vi "Module Template Configuraton Extractor API.vi"(8 "error constant":errorcluster, 11 "data value reference":refnum<data-value>) -> (0 "error out":errorcluster, 3 "Application Config":T1)   [LabVIEW 2021, in "Configuration.lvlib"]
doc: "This method extracts is a Poliphormic method used to read each module configuration."
uses:
  Imposible_Snake_v2/LVApp/Architecture/Modules/Configuration/Configuration.lvlib
  Application/App Configuration.ctl
  Imposible_Snake_v2/LVApp/Modules/Sound Manager/Typedefs/Config.ctl
  Imposible_Snake_v2/LVApp/Modules/Sound Manager/Sound Manager.lvlib
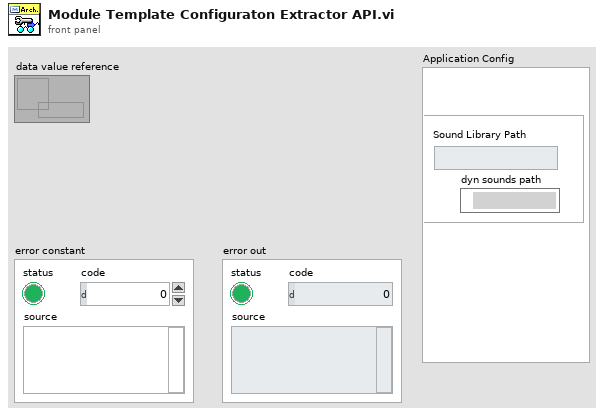
[diagram p1: front panel]
types:
  T1 = typedef "Application.lvclass/App Configuration.ctl" = cluster{"Sound Manager Config":T2}
  T2 = typedef "Sound Manager.lvlib/Config.ctl" = cluster{"Sound Library Path":path, "dyn sounds path":path}
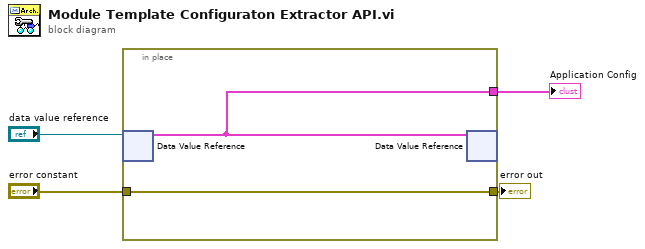
[diagram p0: block diagram]
diagram:
  n1 = in-place {
    in-place-border: [w6] -> w1
    in-place-border: "error constant" -> [w5]
    in-place-border: [w5] -> w2
    n2 = in-place-dvr #1("data value reference") -> (w6:T1)  [unwired: 1 out]
    n3 = in-place-dvr #1(w6) -> ()  [unwired: 2 out]
  }
  "error out" <- w2
  "Application Config" <- w1
